vi "AuMT8852B Output Power Results Query.vi"(8 "error in (no error)":errorcluster, 11 "VISA session":refnum<visa-resource-name>) -> (0 "error out":errorcluster, 2 "error code":i32, 3 "VISA session out":refnum<visa-resource-name>, 4 "Results":T1 {"Test peak power" format="%.2f"; "Packet average; min" format="%.2f"; "Packet average; max" format="%.2f"; "Current packet average power" format="%.2f"})   [LabVIEW 2017]
doc: "Anritsu MT8852B Bluetooth Tester\n\nReturns the results of the Output Power test.\n\nOUTPUTS\nResults - measurements made during the test."
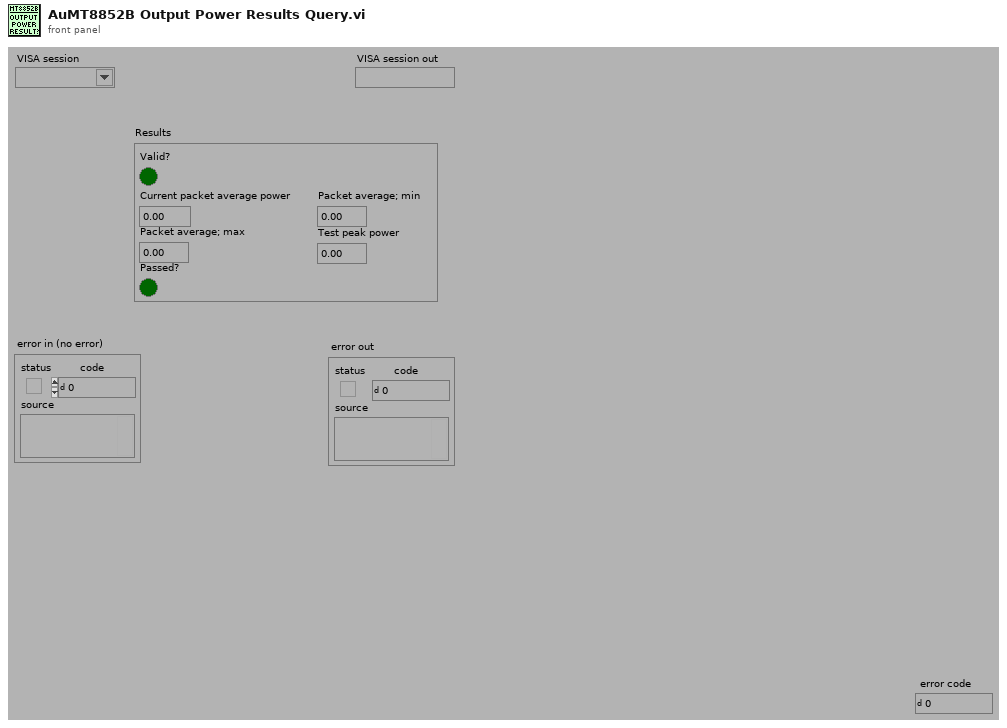
[diagram p1: front panel]
types:
  T1 = cluster{"Valid?":bool, "Current packet average power":dbl, "Packet average; max":dbl, "Packet average; min":dbl, "Test peak power":dbl, "Passed?":bool}
  T2 = enum16{"Simulate", "Range check", "Cache", "Query instrument status"}
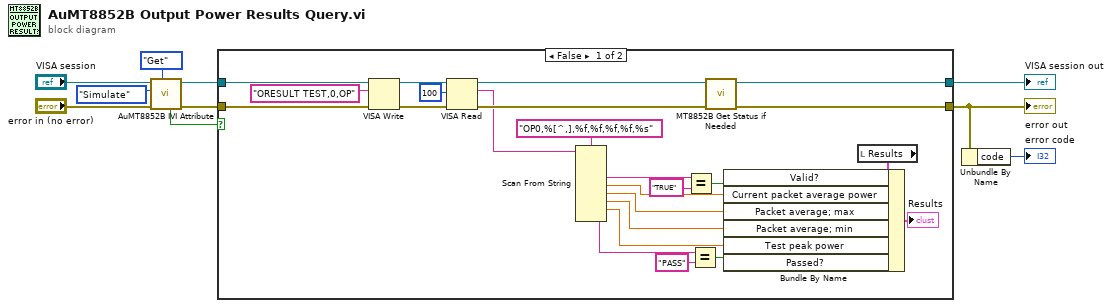
[diagram p0: block diagram]
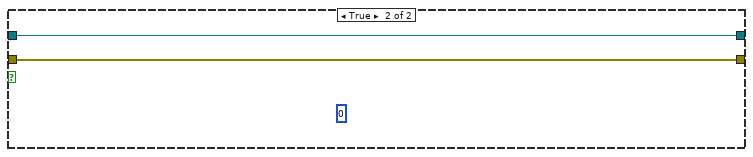
[diagram p2: hidden frame]
diagram:
  n1 = call <instrlib>:"AuMT8852B IVI Attribute.vi"("Set/Get (Set)"=enum16{"Set", "Get"}."Get", "error in (no error)"="error in (no error)", "Flag (Simulate)"=T2."Simulate", "VISA session"="VISA session") -> ("error out"=w7:errorcluster, "VISA session out"=w9:refnum<visa-resource-name>, "Value out"=w3:bool)  [unwired: 5 in]
  n2 = case shown="False" w3 {
    tunnel: [w16 w36] -> w10
    tunnel: [w15 w35] -> w1
    tunnel: w9 -> [w33 w36]
    tunnel: w7 -> [w32 w35]
    frame False {
      n3 = VISA Write(VISA resource name=w33, write buffer="ORESULT TEST,0,OP" ("write buffer (\"\")"), error in (no error)=w32) -> (VISA resource name out=w31:refnum<visa-resource-name>, error out=w30:errorcluster)  [unwired: 1 out]
      n4 = VISA Read(VISA resource name=w31, byte count=u32 100 ("byte count (0)"), error in (no error)=w30) -> (VISA resource name out=w14:refnum<visa-resource-name>, read buffer=w12:string, error out=w13:errorcluster)  [unwired: 1 out]
      n5 = Scan From String(format string="OP0,%[^,],%f,%f,%f,%f,%s" ("Format String"), input string=w12) -> (output 1=w11:string, output 2=w24:dbl, output 3=w23:dbl, output 4=w22:dbl, output 5=w21:dbl, output 6=w18:string)  [unwired: 8 in, 3 out]
      n6 = Equal?(x=w11, y="TRUE") -> (x = y?=w26:bool)
      n7 = Equal?(x=w18, y="PASS") -> (x = y?=w19:bool)
      n8 = call <instrlib>:"MT8852B Get Status if Needed.vi"("error in (no error)"=w13, "VISA session"=w14) -> ("error out"=w15:errorcluster, "VISA session out"=w16:refnum<visa-resource-name>)  [unwired: 8 in]
      n9 = local read "Results"() -> (w27:T1)
      n10 = Bundle By Name(cluster=w27, "Valid?"=w26, "Current packet average power"=w24, "Packet average; max"=w23, "Packet average; min"=w22, "Test peak power"=w21, "Passed?"=w19) -> (→"Results":T1)
    }
    frame True {
      (unwired) u8 0
    }
  }
  "error out" <- w1
  "VISA session out" <- w10
  n11 = Unbundle By Name(w1) -> ("code"=→"error code":i32)
